vi "Contour Line_Preprocess Height Vector.vi"(11 "Height Vector In":dbl[](array[numeric])) -> (3 "Height Vector Out":dbl[](array[numeric]))   [LabVIEW 2020, in "NI_AAL_Geometry.lvlib"]
uses:
  <vilib>/Analysis/NI_AAL_Geometry.lvlib
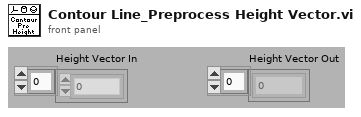
[diagram p1: front panel]
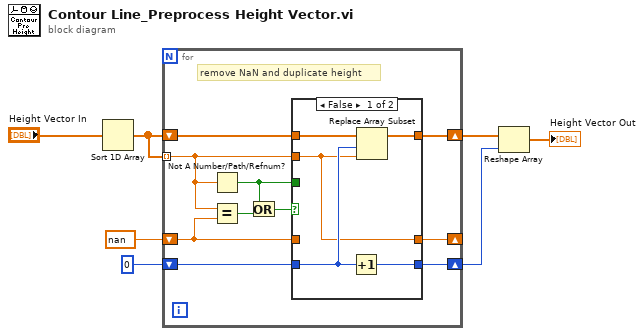
[diagram p0: block diagram]
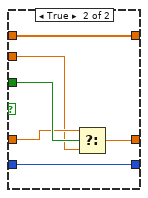
[diagram p2: hidden frame]
diagram:
  n1 = Sort 1D Array(array="Height Vector In") -> (sorted array=w5:dbl[])
  n2 = for {
    shift-right: [w14] -> w2
    shift-left: w5 -> [w17]
    tunnel: w5 -> [w13] mode=indexing
    shift-right: [w10] -> _
    shift-left: nan -> [w8]
    shift-right: [w15] -> w3
    shift-left: 0 -> [w16]
    # "remove NaN and duplicate height"
    n3 = Not A Number/Path/Refnum?(number/path/refnum=w13) -> (NaN/Path/Refnum?=w9:bool)
    n4 = Equal?(x=w13, y=w8) -> (x = y?=w12:bool)
    n5 = Or(x=w9, y=w12) -> (x .or. y?=w11:bool)
    n6 = case shown="False" w11 {
      tunnel: w17 -> [w21 w27]
      tunnel: w16 -> [w20 w28]
      tunnel: [w22 w28] -> w15
      tunnel: w13 -> [w18 w24]
      tunnel: [w19 w27] -> w14
      tunnel: [w18 w23] -> w10
      tunnel: w9 -> [_ w26]
      tunnel: w8 -> [_ w25]
      frame False {
        n7 = Increment(x=w20) -> (x+1=w22:i32)
        n8 = Replace Array Subset(array=w21, new element=w18, index=w20) -> (w19:dbl[])
      }
      frame True {
        n9 = Select(t=w25, s=w26, f=w24) -> (s? t:f=w23:dbl)
      }
    }
  }
  n10 = Reshape Array(w2, w3) -> (→"Height Vector Out":dbl[])
